vi "提取剩余药量信息.vi"(1 "Y变化均值":dbl, 2 "输入ROI（T2）":T1) -> (0 "剩余药量%":dbl)   [LabVIEW 2017]
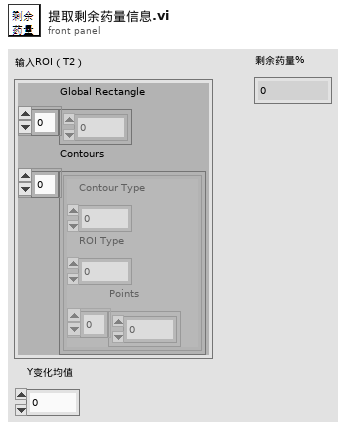
[diagram p1: front panel]
types:
  T1 = cluster{"Global Rectangle":i32[], "Contours":cluster{"Contour Type":u32, "ROI Type":u32, "Points":i32[]}[]}
  T2 = cluster{"Contour Type":u32, "ROI Type":u32, "Points":i32[]}[]
  T3 = cluster{"Contour Type":u32, "ROI Type":u32, "Points":i32[]}
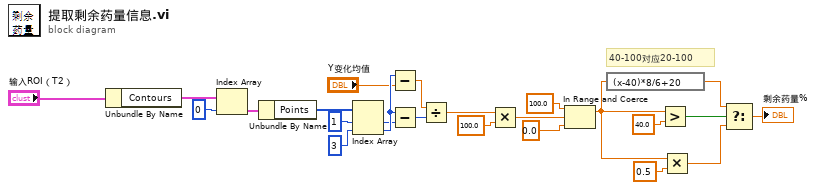
[diagram p0: block diagram]
diagram:
  # "40-100对应20-100"
  n1 = Unbundle By Name("输入ROI（T2）") -> ("Contours"=w23:T2)
  n2 = Index Array(array=w23, index=0 ("索引")) -> (element=w21:T3)
  n3 = Unbundle By Name(w21) -> ("Points"=w20:i32[])
  n4 = Index Array(array=w20, index #1=1, index #2=3) -> (element #1=w16:i32, element #2=w17:i32)
  n5 = Subtract(x=w17, y="Y变化均值") -> (x-y=w19:dbl)
  n6 = Subtract(x=w17, y=w16) -> (x-y=w15:i32)
  n7 = Divide(x=w19, y=w15) -> (x/y=w14:dbl)
  n8 = Multiply(x=w14, y=100.0) -> (x*y=w1:dbl)
  n9 = In Range and Coerce(upper limit=100.0 ("上限"), x=w1, lower limit=0.0 ("上限")) -> (coerced(x)=w3:dbl)  [unwired: 1 out]
  n10 = expression code="(x-40)*8/6+20"(w3) -> (w6:dbl)
  n11 = Greater?(x=w3, y=40.0) -> (0:w7:bool)
  n12 = Multiply(x=w3, y=0.5) -> (x*y=w2:dbl)
  n13 = Select(t=w6, s=w7, f=w2) -> (s? t:f=→"剩余药量%":dbl)
